vi "Untitled 15.vi"() -> ()   [LabVIEW 2011, in "LVH-Adept.lvlib"]
uses:
  <vilib>/LabVIEW Hacker/Adept/LVH-Adept.lvlib
  <vilib>/LabVIEW Hacker/Adept/Private/Type Defs/Adept Device Ctl.xctl
  <vilib>/LabVIEW Hacker/Adept/Private/DPCUTIL/DPCUTIL.lvlib
panel:
  in  "Adept Device":u16(xcontrol)
  in  "Data":u8
  in  "Register Address":u8
  out "Data":u8
  in  "Register Address":u8
  in  "Write Button":bool
  in  "Stop Button":bool
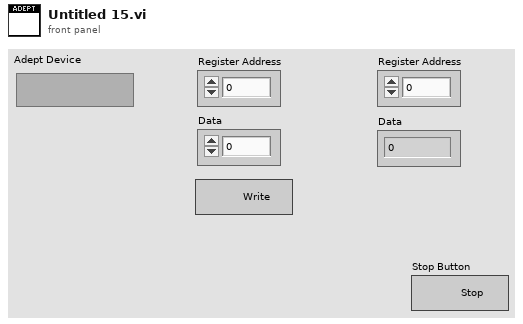
[diagram p1: front panel]
types:
  T1 = typedef "LVH-Adept.lvlib/Device Config.ctl" = cluster{"Num Devices":i32, "Device Names":string[], "Device Index":u16, "Device Handle":u32}
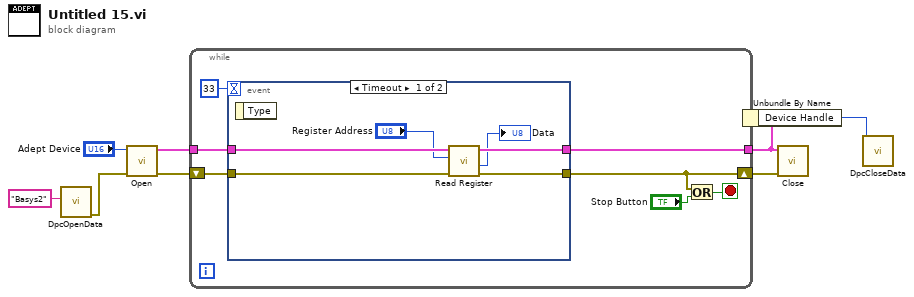
[diagram p0: block diagram]
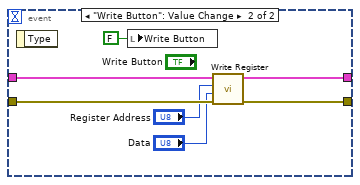
[diagram p2: hidden frame]
diagram:
  n1 = call <vilib>:"DpcOpenData.vi"("Device Name"="Basys2") -> ("Error Out"=w3:errorcluster)  [unwired: 8 in, 2 out]
  n2 = call <vilib>:"Open.vi"("Error In"=w3, "Adept Device Ctl"="Adept Device") -> ("Error Out"=w8:errorcluster, "Adept Config"=w7:T1)  [unwired: 8 in]
  n3 = while {
    tunnel: w7 -> [w14]
    shift-right: [w10] -> w6
    shift-left: w8 -> [w15]
    tunnel: [w11] -> w2
    stop <- w13 stop-if-true
    n4 = event shown="[0] Timeout" {
      selector: _ -> [_ _]
      dyn-events: _ -> [_ _]
      timeout: 33 -> [_ _]
      tunnel: w15 -> [w21 w24]
      tunnel: w14 -> [w20 w25]
      tunnel: [w19 w26] -> w10
      tunnel: [w18 w27] -> w11
      event Timeout {
        n5 = event-data() -> ()  [unwired: 1 in, 1 out]
        n6 = call <vilib>:"Read Register.vi"("Error In"=w21, "Register Address"="Register Address", "Adept Config"=w20) -> ("Error Out"=w19:errorcluster, "Data"=→"Data":u8, "Adept Config"=w18:T1)  [unwired: 6 in]
      }
      event "Write Button": Value Change {
        n7 = event-data() -> ()  [unwired: 1 in, 1 out]
        n8 = local write "Write Button"(FALSE ("Write Button")) -> ()
        n9 = call <vilib>:"Write Register.vi"("Error In"=w24, "Data"="Data", "Register Address"="Register Address", "Adept Config"=w25) -> ("Error Out"=w26:errorcluster, "Adept Config"=w27:T1)  [unwired: 6 in]
      }
    }
    n10 = Or(x=w10, y="Stop Button") -> (x .or. y?=w13:bool)
  }
  n11 = Unbundle By Name(w2) -> ("Device Handle"=w1:u32)
  n12 = call <vilib>:"Close.vi"("Error In"=w6, "Adept Config"=w2) -> ()  [unwired: 9 in, 1 out]
  n13 = call <vilib>:"DpcCloseData.vi"("Device Handle"=w1) -> ()  [unwired: 9 in, 2 out]
